vi "otherprottest.vi"() -> ()   [LabVIEW 2013]
uses:
  domain.ctl
  protocol.ctl
  lvnano.lvlib
panel:
  out "LAST MSG":string
  out "exectime":dbl
  in  "messages":i32=1
  in  "size":i32=1024
  out "error out":errorcluster
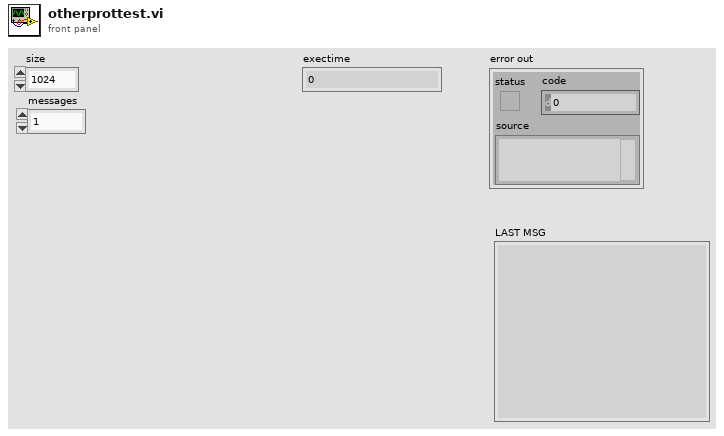
[diagram p1: front panel]
types:
  T1 = typedef "lvnano.lvlib/protocol.ctl" = i32
  T2 = typedef "lvnano.lvlib/domain.ctl" = enum16{"Invalid", "AF_SP", "AF_SP_RAW"}
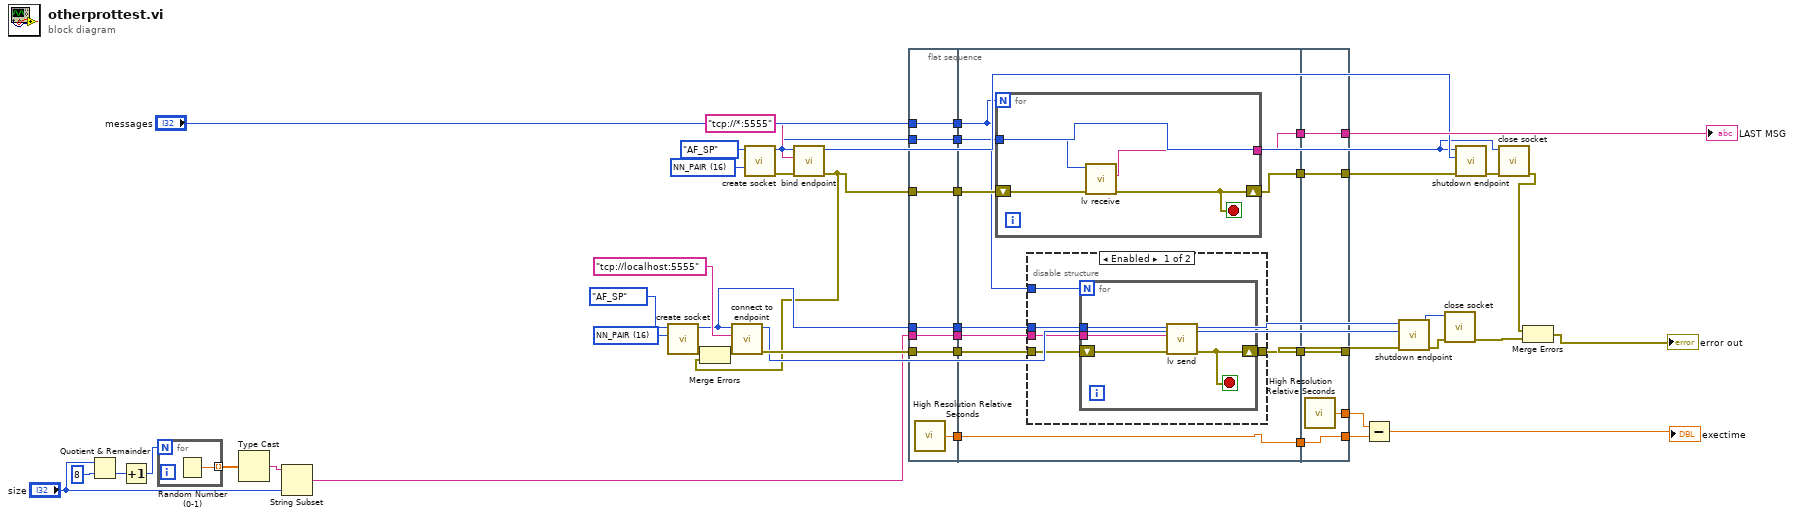
[diagram p0: block diagram]
diagram:
  w2 = T1 16 items=["NN_PUSH"=80, "NN_PULL"=81, "NN_BUS"=112, "NN_PAIR"=16, "NN_PUB"=32, "NN_SUB"=33, "NN_REQ"=48, "NN_REP"=49, "NN_SURVEYOR"=96, "NN_RESPONDENT"=97] ("protocol")
  w3 = T1 16 items=["NN_PUSH"=80, "NN_PULL"=81, "NN_BUS"=112, "NN_PAIR"=16, "NN_PUB"=32, "NN_SUB"=33, "NN_REQ"=48, "NN_REP"=49, "NN_SURVEYOR"=96, "NN_RESPONDENT"=97] ("protocol")
  n1 = Quotient & Remainder(x="size", y=8) -> (floor(x/y)=w44:i32)  [unwired: 1 out]
  n2 = Increment(x=w44) -> (x+1=w42:i32)
  n3 = for {
    N: w42 -> [_]
    tunnel: [w46] -> w41 mode=indexing
    n4 = Random Number (0-1)() -> (number: 0 to 1=w46:dbl)
  }
  n5 = Type Cast(x=w41) -> (*(type *) &x=w40:string)  [unwired: 1 in]
  n6 = String Subset(string=w40, length (rest)="size") -> (substring=w1:string)  [unwired: 1 in]
  n7 = call "create socket.vi"("protocol"=w2, "domain"=domain."AF_SP") -> ("error out"=w20:errorcluster, "socket"=w15:i64)  [unwired: 8 in]
  n8 = call "create socket.vi"("protocol"=w3, "domain"=domain."AF_SP") -> ("error out"=w24:errorcluster, "socket"=w9:i64)  [unwired: 8 in]
  n9 = call "bind endpoint.vi"("error in"=w24, "address"="tcp://*:5555" ("addr"), "socket"=w9) -> ("error out"=w4:errorcluster, "endpoint"=w10:i32)  [unwired: 7 in]
  n10 = Merge Errors(w20, w4) -> (w5:errorcluster)
  n11 = call "connect to endpoint.vi"("error in"=w5, "address"="tcp://localhost:5555" ("addr"), "socket"=w15) -> ("error out"=w18:errorcluster, "endpoint"=w11:i32)  [unwired: 7 in]
  n12 = flat-sequence {
    tunnel: w1 -> [w48]
    tunnel: "messages" -> [w49]
    tunnel: w9 -> [w50]
    tunnel: w15 -> [w51]
    tunnel: w18 -> [w52]
    tunnel: w4 -> [w53]
    tunnel: [w53] -> w35
    tunnel: [w52] -> w34
    tunnel: [w51] -> w33
    tunnel: [w50] -> w32
    tunnel: [w49] -> w31
    tunnel: [w48] -> w30
    tunnel: [w47] -> w29
    tunnel: [w61] -> w28
    tunnel: [w58] -> w27
    tunnel: w35 -> [w63]
    tunnel: w34 -> [w62]
    tunnel: w33 -> [w60]
    tunnel: w32 -> [w59]
    tunnel: w31 -> [w55]
    tunnel: w30 -> [w57]
    tunnel: w29 -> [w56]
    tunnel: [w56] -> w26
    tunnel: [w54] -> w25
    tunnel: [w81] -> w8
    tunnel: [w82] -> w17
    tunnel: w28 -> [w82]
    tunnel: w27 -> [w81]
    tunnel: [w80] -> w7
    tunnel: w26 -> [w79]
    tunnel: [w79] -> w6
    tunnel: w25 -> [w78]
    tunnel: [w78] -> w36
    frame #0 {
      n13 = call <vilib>:"High Resolution Relative Seconds.vi"() -> ("relative seconds"=w47:dbl)
    }
    frame #1 {
      n14 = for {
        N: w55 -> [_]
        tunnel: w59 -> [w76]
        shift-right: [w75] -> w58
        shift-left: w63 -> [w77]
        tunnel: [w74] -> w54
        stop <- w75 stop-if-true
        n15 = call "lv receive.vi"("error in"=w77, "socket"=w76) -> ("error out"=w75:errorcluster, "data"=w74:string)  [unwired: 8 in]
      }
      n16 = disable-structure shown="Enabled" {
        disable-tunnel: w62 -> [w68 w73]
        disable-tunnel: [w67 w73] -> w61
        disable-tunnel: w60 -> [w66 _]
        disable-tunnel: w57 -> [w65 _]
        disable-tunnel: w55 -> [w64 _]
        frame Enabled {
          n17 = for {
            N: w64 -> [_]
            tunnel: w65 -> [w71]
            tunnel: w66 -> [w70]
            shift-right: [w69] -> w67
            shift-left: w68 -> [w72]
            stop <- w69 stop-if-true
            n18 = call "lv send.vi"("error in"=w72, "data"=w71, "socket"=w70) -> ("error out"=w69:errorcluster)  [unwired: 8 in]
          }
        }
        frame Disabled {
        }
      }
    }
    frame #2 {
      n19 = call <vilib>:"High Resolution Relative Seconds.vi"() -> ("relative seconds"=w80:dbl)
    }
  }
  n20 = Subtract(x=w7, y=w6) -> (x-y=→"exectime":dbl)
  n21 = call "shutdown endpoint.vi"("error in"=w17, "endpoint"=w11, "socket"=w15) -> ("error out"=w14:errorcluster)  [unwired: 8 in]
  n22 = call "close socket.vi"("error in"=w14, "socket"=w15) -> ("error out"=w12:errorcluster)  [unwired: 9 in]
  n23 = call "shutdown endpoint.vi"("error in"=w8, "endpoint"=w10, "socket"=w9) -> ("error out"=w16:errorcluster)  [unwired: 8 in]
  n24 = call "close socket.vi"("error in"=w16, "socket"=w9) -> ("error out"=w13:errorcluster)  [unwired: 9 in]
  n25 = Merge Errors(w13, w12) -> (→"error out":errorcluster)
  "LAST MSG" <- w36
